vi "Init Drive Motors With CVS File.vi"() -> ()   [LabVIEW 2018]
uses:
  <vilib>/Rock Robotics/WPI/RobotDrive/WPI_RobotDriveOpen4MotorWithExistingMotors.vi
  <vilib>/Rock Robotics/WPI/RobotDrive/WPI_RobotDriveOpen2MotorWithExistingMotors.vi
  <vilib>/Rock Robotics/WPI/MotorControl/WPI_MotorControlOpen Jaguar.vi
panel:
  out "Grpper PWM":u8
  out "Drive Right Front":u8
  out "Drive Left Front":i32
  out "Drive Right Rear":i32
  out "Drive Left Rear":u8
  out "Drive Right Center":u8
  out "Drive Left Center":i32
  out "Arm Shoulder":u8
  out "Arm Base":u8
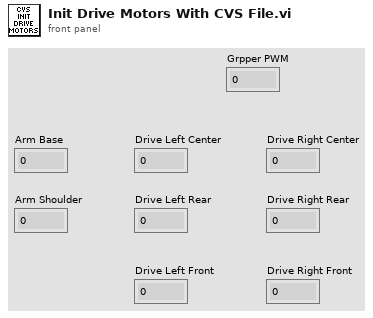
[diagram p1: front panel]
types:
  T1 = typedef "WPI_MotorControlDeviceRef.ctl" = cluster{"DeviceStatus":errorcluster, "Type":T2, "PWM":cluster{"PWM Channel":T3, "DeadBand":T4}, "CAN":cluster{"Device Number":u8, "SetOutput VI Ref":variant, "GetOutput VI Ref":variant, "Enable VI Ref":variant, "Disable VI Ref":variant, "Data":variant}, "Invert":bool, "DIO PWM":cluster{"PWM \"Enable\" Channel":T3, "DIOChannel":T5, "PWM Rate":dbl}}
  T2 = typedef "WPI_MotorControlType.ctl" = enum16{"PWM", "CAN", "DIO PWM"}
  T3 = typedef "FPGA_DIOPWMChannel.ctl" = enum8{"PWM 0", "PWM 1", "PWM 2", "PWM 3", "PWM 4", "PWM 5", "PWM 6", "PWM 7", "PWM 8", "PWM 9", "PWM MXP 0", "PWM MXP 1", "PWM MXP 2", "PWM MXP 3", "PWM MXP 4", "PWM MXP 5", "PWM MXP 6", "PWM MXP 7", "PWM MXP 8", "PWM MXP 9", "Invalid"}
  T4 = typedef "WPI_PWMDeadband.ctl" = cluster{"Name":string, "maxPositivePwm":i32, "minPositivePwm":i32, "centerPwm":i32, "maxNegativePwm":i32, "minNegativePwm":i32, "angularRange":u16}
  T5 = typedef "FPGA_DIOChannel.ctl" = enum8{"DIO 0", "DIO 1", "DIO 2", "DIO 3", "DIO 4", "DIO 5", "DIO 6", "DIO 7", "DIO 8", "DIO 9", "DIO MXP 0", "DIO MXP 1", "DIO MXP 2", "DIO MXP 3", "DIO MXP 4", "DIO MXP 5", "DIO MXP 6", "DIO MXP 7", "DIO MXP 8", "DIO MXP 9", "DIO MXP 10", "DIO MXP 11", "DIO MXP 12", "DIO MXP 13", "DIO MXP 14", "DIO MXP 15", "SPI Port CS1", "SPI Port CS2", "SPI Port CS3", "SPI Port MISO", "SPI Port MOSI", "Invalid"}
  T6 = typedef "WPI_RobotDriveDevRef.ctl" = cluster{"DevStatus":errorcluster, "Motors[]":T1[], "Square Inputs":bool, "Max Output":dbl}
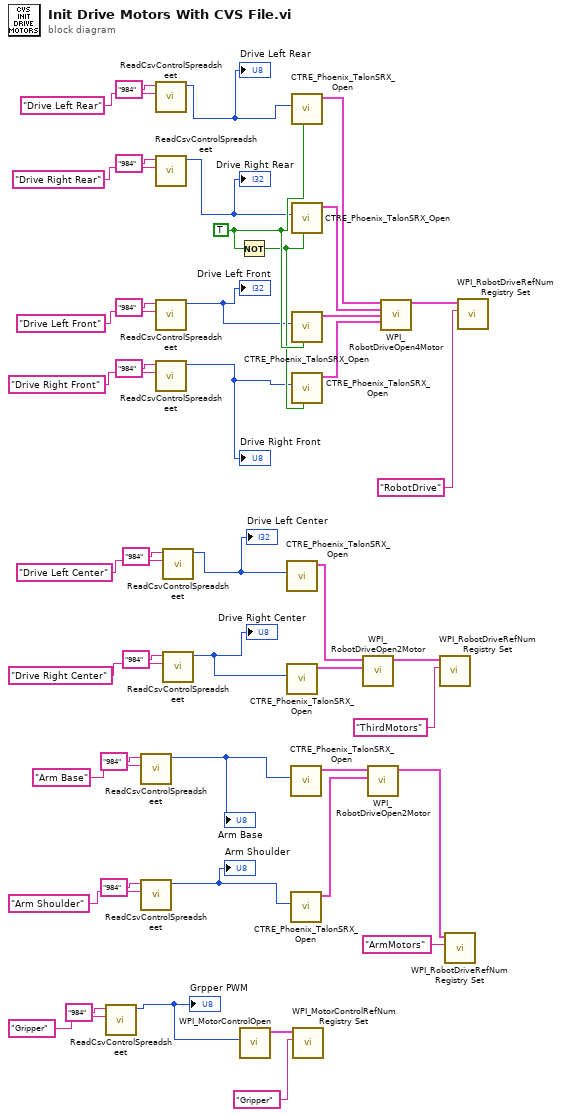
[diagram p0: block diagram]
diagram:
  w39 = TRUE ("Invert")
  n1 = call "ReadCsvControlSpreadsheet.vi"("Motor ID"="Gripper", "Robot ID"="984") -> ("Can Bus ID"=w5:u8)  [unwired: 1 in, 8 out]
  "Grpper PWM" <- w5
  n2 = call "ReadCsvControlSpreadsheet.vi"("Motor ID"="Arm Base", "Robot ID"="984") -> ("Can Bus ID"=w3:u8)  [unwired: 1 in, 8 out]
  "Arm Base" <- w3
  n3 = call "ReadCsvControlSpreadsheet.vi"("Motor ID"="Arm Shoulder", "Robot ID"="984") -> ("Can Bus ID"=w4:u8)  [unwired: 1 in, 8 out]
  "Arm Shoulder" <- w4
  n4 = call "ReadCsvControlSpreadsheet.vi"("Motor ID"="Drive Left Rear", "Robot ID"="984") -> ("Can Bus ID"=w8:u8)  [unwired: 1 in, 8 out]
  "Drive Left Rear" <- w8
  n5 = call "ReadCsvControlSpreadsheet.vi"("Motor ID"="Drive Right Rear", "Robot ID"="984") -> ("Can Bus ID"=w9:u8)  [unwired: 1 in, 8 out]
  "Drive Right Rear" <- w9
  n6 = call "ReadCsvControlSpreadsheet.vi"("Motor ID"="Drive Left Front", "Robot ID"="984") -> ("Can Bus ID"=w7:u8)  [unwired: 1 in, 8 out]
  "Drive Left Front" <- w7
  n7 = call "ReadCsvControlSpreadsheet.vi"("Motor ID"="Drive Right Front", "Robot ID"="984") -> ("Can Bus ID"=w6:u8)  [unwired: 1 in, 8 out]
  "Drive Right Front" <- w6
  n8 = call "ReadCsvControlSpreadsheet.vi"("Motor ID"="Drive Left Center", "Robot ID"="984") -> ("Can Bus ID"=w1:u8)  [unwired: 1 in, 8 out]
  "Drive Left Center" <- w1
  n9 = call "ReadCsvControlSpreadsheet.vi"("Motor ID"="Drive Right Center", "Robot ID"="984") -> ("Can Bus ID"=w2:u8)  [unwired: 1 in, 8 out]
  "Drive Right Center" <- w2
  n10 = Not(x=w39) -> (.not. x?=w38:bool)
  n11 = call-poly <vilib>:"WPI_MotorControlOpen.vi"("PWM Channel"=w5) -> ("MotorControlDeviceRef"=w11:T1)  [unwired: 9 in, 1 out]
  n12 = call <vilib>:"CTRE_Phoenix_TalonSRX_Open.vi"("Device Number"=w1) -> ("CAN Talon SRX Ref"=w37:T1)  [unwired: 9 in, 1 out]
  n13 = call <vilib>:"CTRE_Phoenix_TalonSRX_Open.vi"("Device Number"=w2) -> ("CAN Talon SRX Ref"=w36:T1)  [unwired: 9 in, 1 out]
  n14 = call <vilib>:"CTRE_Phoenix_TalonSRX_Open.vi"("Device Number"=w3) -> ("CAN Talon SRX Ref"=w33:T1)  [unwired: 9 in, 1 out]
  n15 = call <vilib>:"CTRE_Phoenix_TalonSRX_Open.vi"("Device Number"=w4) -> ("CAN Talon SRX Ref"=w32:T1)  [unwired: 9 in, 1 out]
  n16 = call <vilib>:"CTRE_Phoenix_TalonSRX_Open.vi"("Invert"=w39, "Device Number"=w8) -> ("CAN Talon SRX Ref"=w43:T1)  [unwired: 8 in, 1 out]
  n17 = call <vilib>:"CTRE_Phoenix_TalonSRX_Open.vi"("Invert"=w38, "Device Number"=w9) -> ("CAN Talon SRX Ref"=w42:T1)  [unwired: 8 in, 1 out]
  n18 = call <vilib>:"CTRE_Phoenix_TalonSRX_Open.vi"("Invert"=w39, "Device Number"=w7) -> ("CAN Talon SRX Ref"=w41:T1)  [unwired: 8 in, 1 out]
  n19 = call <vilib>:"CTRE_Phoenix_TalonSRX_Open.vi"("Invert"=w38, "Device Number"=w6) -> ("CAN Talon SRX Ref"=w40:T1)  [unwired: 8 in, 1 out]
  n20 = call <vilib>:"WPI_MotorControlRefNum Registry Set.vi"("refnum name"="Gripper", "MotorControlDevRef"=w11) -> ()  [unwired: 8 in, 2 out]
  n21 = call-poly <vilib>:"WPI_RobotDriveOpen2Motor.vi"("Right Motor Dev Ref"=w36, "Left Motor Dev Ref"=w37) -> ("RobotDriveDevRef"=w35:T6)  [unwired: 8 in, 1 out]
  n22 = call-poly <vilib>:"WPI_RobotDriveOpen2Motor.vi"("Right Motor Dev Ref"=w32, "Left Motor Dev Ref"=w33) -> ("RobotDriveDevRef"=w31:T6)  [unwired: 8 in, 1 out]
  n23 = call-poly <vilib>:"WPI_RobotDriveOpen4Motor.vi"("Rear Left Motor Dev Ref"=w43, "Rear Right Motor Dev Ref"=w42, "Front Left Motor Dev Ref"=w41, "Front Right Motor Dev Ref"=w40) -> ("RobotDriveDevRef"=w44:T6)  [unwired: 10 in, 1 out]
  n24 = call <vilib>:"WPI_RobotDriveRefNum Registry Set.vi"("refnum name"="ThirdMotors", "RobotDriveDevRef"=w35) -> ()  [unwired: 8 in, 2 out]
  n25 = call <vilib>:"WPI_RobotDriveRefNum Registry Set.vi"("refnum name"="ArmMotors", "RobotDriveDevRef"=w31) -> ()  [unwired: 8 in, 2 out]
  n26 = call <vilib>:"WPI_RobotDriveRefNum Registry Set.vi"("refnum name"="RobotDrive", "RobotDriveDevRef"=w44) -> ()  [unwired: 8 in, 2 out]
